vi "gps.vi"(4 "error in":errorcluster, 7 "GPS Configuration":string=" {\n \t\"type\": \"GPS\",\n \t\"listen_port\": 8400,\n \t\"location\": {\n \t\t\"x\": 30.0,\n \t\t\"y\": 0.0,\n \t\t\"z\": 110.0\n \t},\n \t\"rotation\": {\n \t\t\"pitch\": 0.0,\n \t\t\"yaw\": 0.0,\n \t\t\"roll\": 0.0\n \t},\n \t\"anchor_overrides\": {\n \t\t\"use_override\": false,\n \t\t\"gis_anchor\": [-90.0, 30.0, 0.0],\n \t\t\"world_anchor\": [0.0, 0.0, 0.0],\n \t\t\"rotation\": -90\n \t}\n }") -> (0 "error out":errorcluster, 1 "GPS Configuration":string, 2 "Raw data":string, 3 "GPS Sample":T2 {"forward"."forward z" format="%#_3g"; "forward"."forward y" format="%#_3g"; "forward"."forward x" format="%#_3g"; "ego_yaw" format="%#_3g"; "ego_speed" format="%#.3f"; "WorldLocation_x" format="%#_3g"; "WorldLocation_y" format="%#_3g"; "latitude" format="%#_3g"; "longitude" format="%#_3g"; "elevation" format="%#_3g"})   [LabVIEW 2019, in "Lib_Simx.lvlib"]
doc: "Configure and reads the data stream for the GPS sensor."
uses:
  Lib_Simx.lvlib
  tools/simx_common.vi
  controls/gps_packet.ctl
  controls/Header.ctl
panel:
  out "Header":T1
  in  "Show Map":bool
  out "Map":picture
  out "Speed":sgl(knob) scale=0.0..200.0
  in  "null connection":refnum<k5>
  # "km/hr"
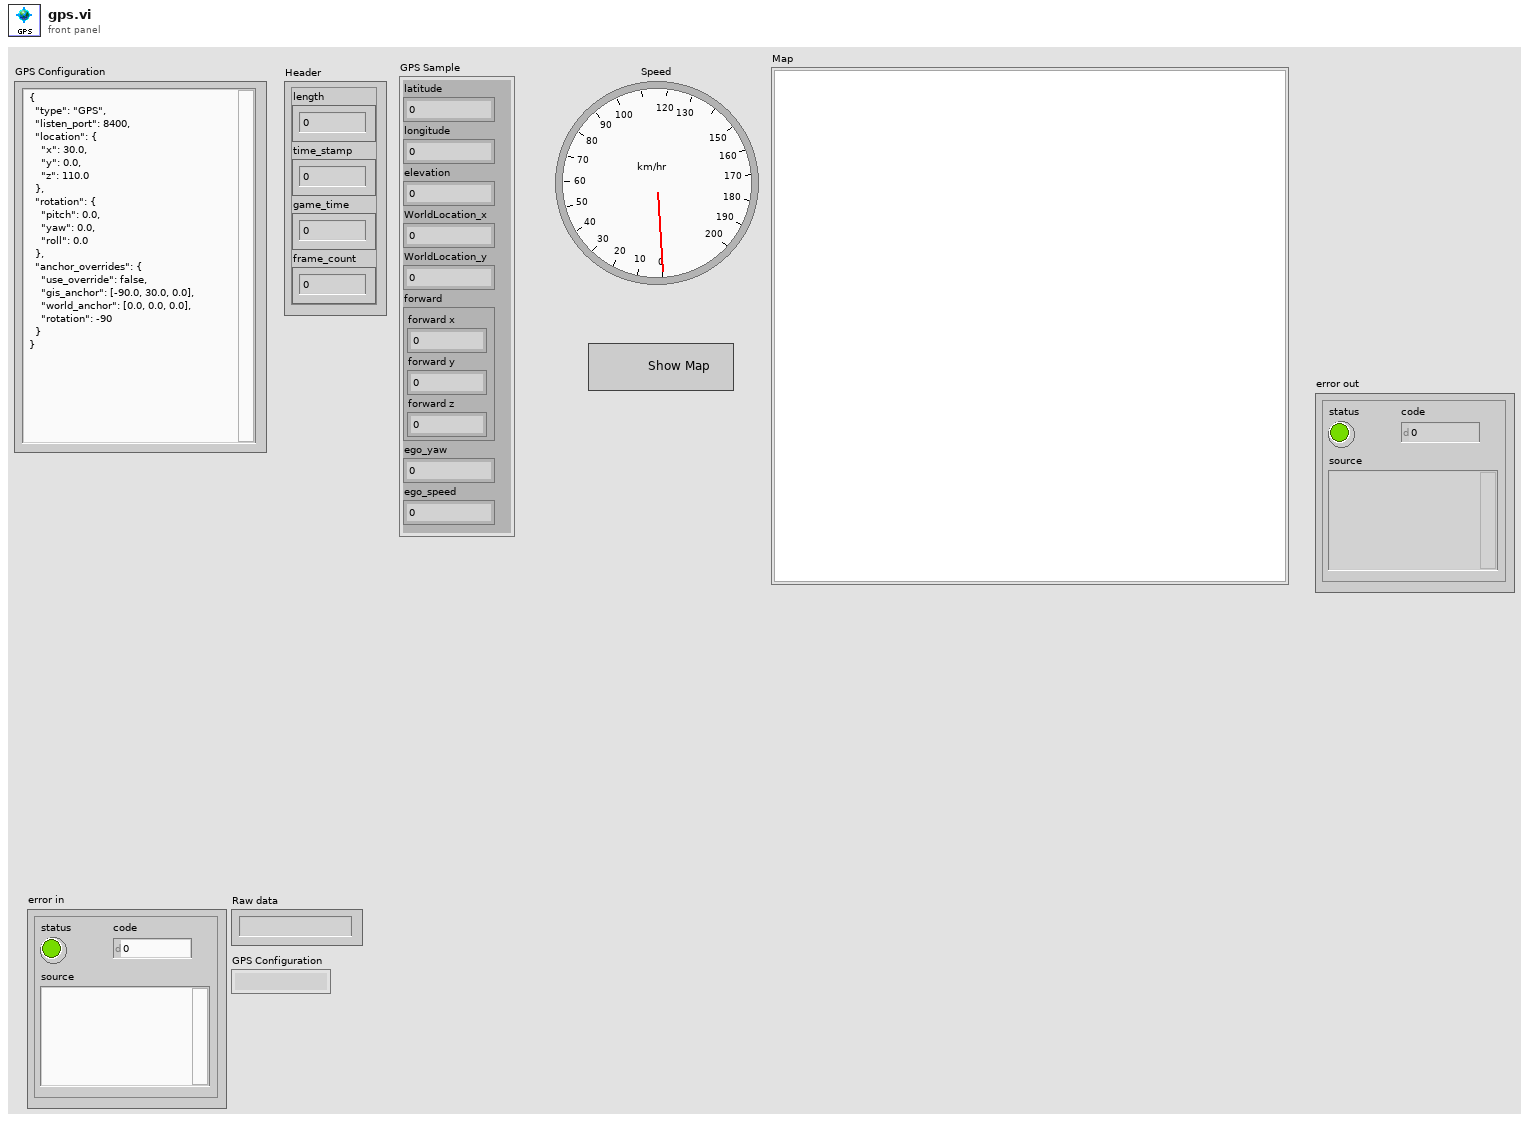
[diagram p1: front panel]
types:
  T1 = typedef "Lib_Simx.lvlib/Header.ctl" = cluster{"length":u32, "time_stamp":u32, "game_time":sgl, "frame_count":u32}
  T2 = typedef "Lib_Simx.lvlib/gps_packet.ctl" = cluster{"latitude":dbl, "longitude":dbl, "elevation":dbl, "WorldLocation_x":sgl, "WorldLocation_y":sgl, "forward":cluster{"forward x":sgl, "forward y":sgl, "forward z":sgl}, "ego_yaw":sgl, "ego_speed":sgl, "horizontal_accuracy":u16, "vertical_accuracy":u16, "satellites":u8, "mode":u8, "CRC":u16}
  T3 = typedef "Lib_Simx.lvlib/simx_connection.ctl" = cluster{"Config":T4, "Connections":T7, "Map":cluster{"lanes":cluster{"x":dbl[], "y":dbl[], "z":dbl[]}, "StartPosition":cluster{"start_points":T8, "StartRotation":dbl[], "StartLocation":dbl[]}, "Draw Map Size":T9, "DrawArea":cluster{"min_Y":dbl, "min_X":dbl, "Scale X":dbl, "Scale Y":dbl}, "Map":picture, "Map Geojson":string}}
  T4 = typedef "Lib_Simx.lvlib/config.ctl" = cluster{"Trajectory":T5, "Weather":T6}
  T5 = typedef "Lib_Simx.lvlib/trajectory.ctl" = cluster{"Number of frames":i32, "Frame number":i32, "Trajectory":string}
  T6 = typedef "Lib_Simx.lvlib/weather.ctl" = cluster{"id":string}
  T7 = typedef "Lib_Simx.lvlib/connections.ctl" = cluster{"Simulator Connection":refnum<k5>, "server_ip":string, "Port":i32, "Sensor connections":refnum<k5>[]}
  T8 = typedef "Lib_Simx.lvlib/start_points.ctl" = cluster{"locations":dbl[][], "rotations":dbl[][], "type":string[]}
  T9 = typedef "LVBoundsTypeDef.ctl" = cluster{"Width":u32, "Height":u32}
  T10 = enum16{"big-endian, network order", "native, host order", "little-endian"}
  T11 = cluster{"Width":u16, "Style":enum32{"Solid", "Dash", "Dot", "DashDot", "DashDotDot"}}
  T12 = typedef "Lib_Simx.lvlib/sensor_sample.ctl" = cluster{"Header":T1, "data out":string}
  T13 = cluster{"lanes":cluster{"x":dbl[], "y":dbl[], "z":dbl[]}, "StartPosition":cluster{"start_points":T8, "StartRotation":dbl[], "StartLocation":dbl[]}, "Draw Map Size":T9, "DrawArea":cluster{"min_Y":dbl, "min_X":dbl, "Scale X":dbl, "Scale Y":dbl}, "Map":picture, "Map Geojson":string}
  T14 = cluster{"min_Y":dbl, "min_X":dbl, "Scale X":dbl, "Scale Y":dbl}
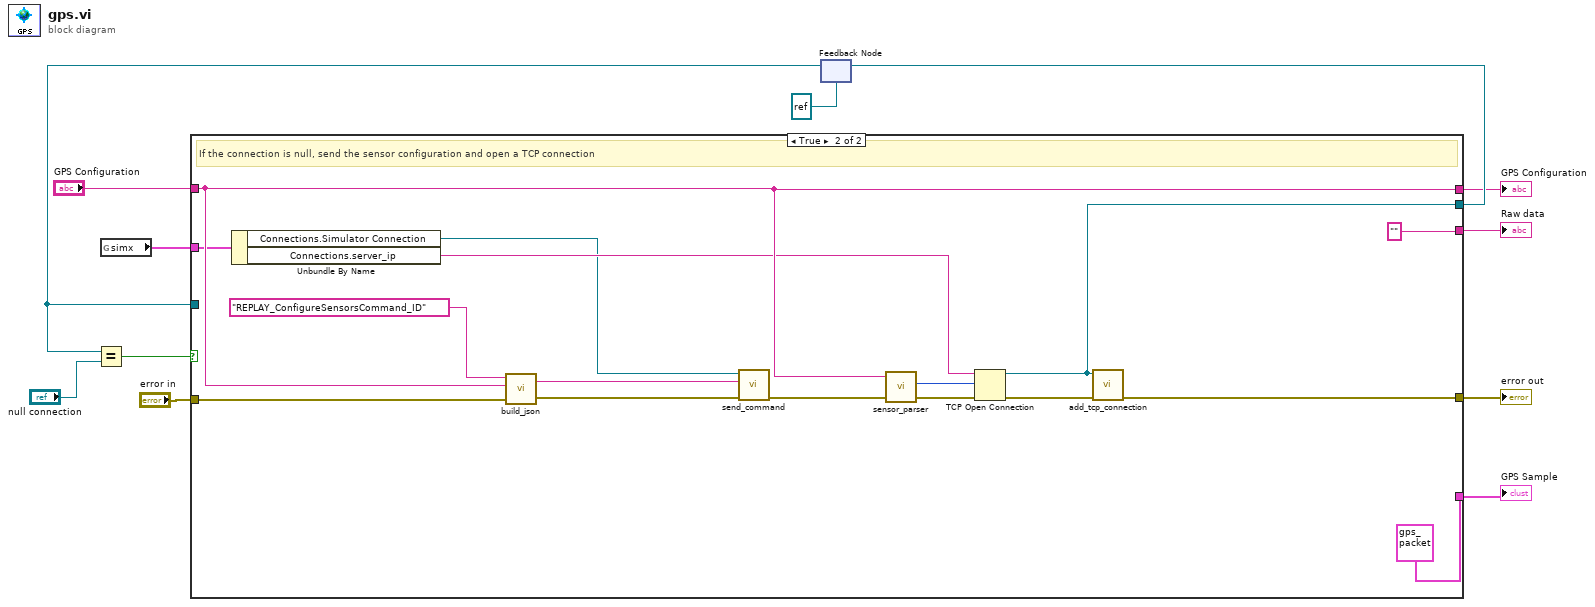
[diagram p0: block diagram]
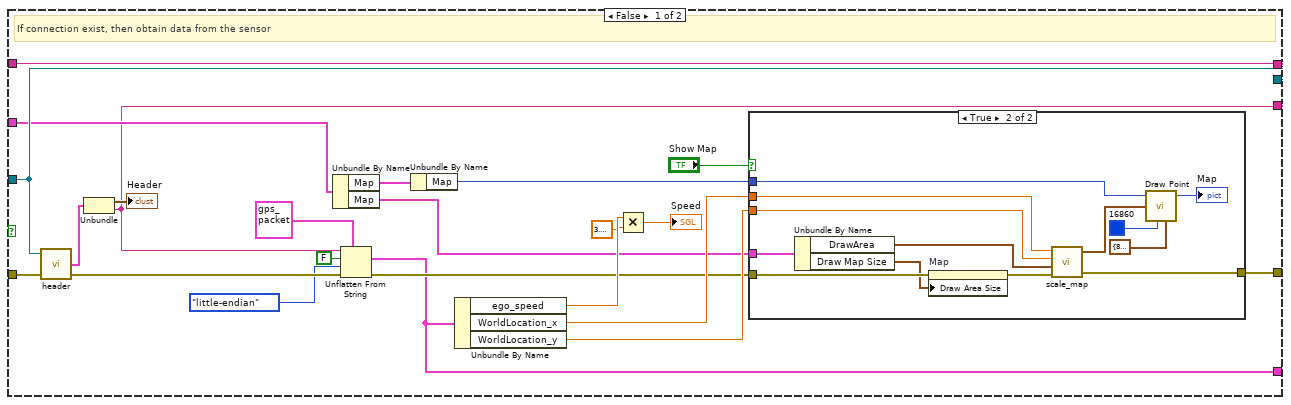
[diagram p2: hidden frame]
diagram:
  n1 = global read "simx_common.vi" "simx"() -> (w3:T3)
  n2 = feedback #1(refnum<k5> refnum ("connection ID")) -> (w8:refnum<k5>)
  n3 = Equal?(x=w8, y="null connection") -> (x = y?=w9:bool)
  n4 = case shown="True" w9 {
    tunnel: [w16 w58] -> w6
    tunnel: "GPS Configuration" -> [w29 w55]
    tunnel: [w30 w57] -> w10
    tunnel: w8 -> [w30 _]
    tunnel: "error in" -> [w31 w60]
    tunnel: [w14 "" ("data out")] -> w5
    tunnel: [w29 w55] -> w4
    tunnel: w3 -> [w21 w53]
    tunnel: [w13 T2 {"latitude"=0.0, "longitude"=0.0, "elevation"=0.0, "WorldLocation_x"=0.0, "WorldLocation_y"=0.0, "forward"={"forward x"=0.0, "forward y"=0.0, "forward z"=0.0}, "ego_yaw"=0.0, "ego_speed"=0.0, "horizontal_accuracy"=0, "vertical_accuracy"=0, "satellites"=0, "mode"=0, "CRC"=0} ("GPS Sample")] -> w1
    frame False {
      # "If connection exist, then obtain data from the sensor"
      n5 = call "header.vi"("error in"=w31, "TCP Network Connection in"=w30) -> ("error out"=w34:errorcluster, "Sensor sample"=w35:T12)  [unwired: 1 in, 1 out]
      n6 = Unbundle(w35) -> ("Header"=→"Header":T1, "data out"=w14:string)
      n7 = Unbundle By Name(w21) -> ("Map"=w19:T13, "Map"=w20:T13)
      n8 = Unflatten From String(type=T2 {"latitude"=0.0, "longitude"=0.0, "elevation"=0.0, "WorldLocation_x"=0.0, "WorldLocation_y"=0.0, "forward"={"forward x"=0.0, "forward y"=0.0, "forward z"=0.0}, "ego_yaw"=0.0, "ego_speed"=0.0, "horizontal_accuracy"=0, "vertical_accuracy"=0, "satellites"=0, "mode"=0, "CRC"=0} ("gps format"), binary string=w14, data includes array or string size? (T)=FALSE, byte order (0:big-endian, network order)=T10."little-endian", error in (no error)=w34) -> (value=w13:T2, error out=w17:errorcluster)  [unwired: 1 out]
      n9 = Unbundle By Name(w19) -> ("Map"=w18:picture)
      n10 = Unbundle By Name(w13) -> ("ego_speed"=w28:sgl, "WorldLocation_x"=w25:sgl, "WorldLocation_y"=w24:sgl)
      n11 = Multiply(x=w28, y=sgl 3.6) -> (x*y=→"Speed":sgl)
      n12 = case shown="True" "Show Map" {
        tunnel: w25 -> [_ w39]
        tunnel: w24 -> [_ w38]
        tunnel: w18 -> [_ w46]
        tunnel: w17 -> [w36 w43]
        tunnel: [w36 w44] -> w16
        tunnel: w20 -> [_ w42]
        frame False {
        }
        frame True {
          n13 = Unbundle By Name(w42) -> ("DrawArea"=w40:T14, "Draw Map Size"=w41:T9)
          n14 = property on="Map" class="Pict"(error in=w43, "Draw Area Size"=w41) -> (error out=w37:errorcluster)  [unwired: 1 in, 1 out]
          n15 = call "scale_map.vi"("error in"=w37, "Map.DrawArea"=w40, "location y"=w38, "location x"=w39) -> ("error out"=w44:errorcluster, "point(x,y)"=w47:cluster{"x":i16, "y":i16})  [unwired: 1 in]
          n16 = call <vilib>:"Draw Point.vi"("picture"=w46, "point(x,y)"=w47, "color(black)"=u32 16860, "pen"=T11 {"Width"=8, "Style"=enum."Solid"}) -> ("new picture"=→"Map":picture)  [unwired: 5 in]
        }
      }
    }
    frame True {
      # "If the connection is null, send the sensor configuration and open a TCP connection"
      n17 = Unbundle By Name(w53) -> ("Connections.Simulator Connection"=w51:refnum<k5>, "Connections.server_ip"=w52:string)
      n18 = call "build_json.vi"("error in"=w60, "Message"=w55, "Command_ID"="REPLAY_ConfigureSensorsCommand_ID") -> ("error out"=w63:errorcluster, "JSON Out"=w64:string)  [unwired: 1 in]
      n19 = call "send_command.vi"("error in"=w63, "JSON Command"=w64, "TCP Network Connection in"=w51) -> ("error out"=w62:errorcluster)  [unwired: 1 in, 3 out]
      n20 = call "sensor_parser.vi"("Sensor configuration"=w55, "error in"=w62) -> ("Port out"=w54:u16, "error out"=w56:errorcluster)  [unwired: 1 in, 2 out]
      n21 = TCP Open Connection(address=w52, remote port or service name=w54, error in (no error)=w56) -> (connection ID=w57:refnum<k5>, error out=w61:errorcluster)  [unwired: 2 in]
      n22 = call "add_tcp_connection.vi"("error in"=w61, "Sensor connection"=w57) -> ("error out"=w58:errorcluster)  [unwired: 5 in]
    }
  }
  "error out" <- w6
  "Raw data" <- w5
  "GPS Configuration" <- w4
  "GPS Sample" <- w1
  n23 = feedback-in #1(w10) -> ()
